vi "General Format send.vi"() -> ()   [LabVIEW 2009]
panel:
  out "VISA resource name out":refnum<visa-resource-name>
  out "error out":errorcluster
  in  "error in (no error)":errorcluster
  in  "VISA resource name":refnum<visa-resource-name>="GPIB0::21::INSTR"
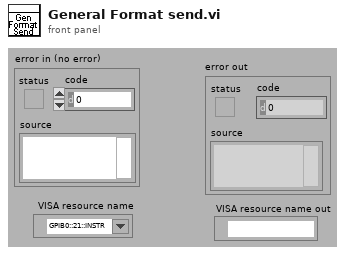
[diagram p1: front panel]
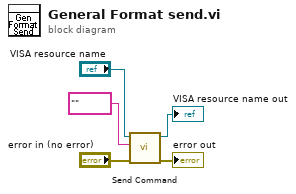
[diagram p0: block diagram]
diagram:
  n1 = call "Send Command.vi"("error in (no error)"="error in (no error)", "write buffer"="", "VISA resource name"="VISA resource name") -> ("error out"=→"error out":errorcluster, "VISA resource name out"=→"VISA resource name out":refnum<visa-resource-name>)  [unwired: 7 in]
